vi "Excel Get Last Row (dynamic wrapper).vi"(0 "report in":refnum<class "NI_report.lvclass">, 7 "offset":i32, 11 "error in (no error)":errorcluster, 12 "MS Office parameters":T1) -> (4 "report out":refnum<class "NI_report.lvclass">, 14 "MS Office parameters out":T1, 15 "error out":errorcluster)   [LabVIEW 2020, in "NI_ReportGenerationCore.lvlib"]
uses:
  <vilib>/Utility/NIReport.llb/NI_ReportGenerationCore.lvlib
  <vilib>/Utility/NIReport.llb/NI_report.lvclass
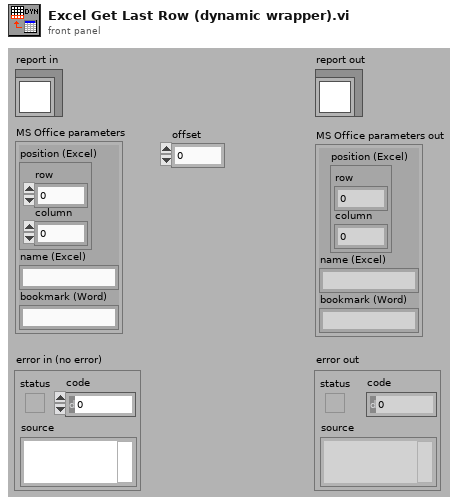
[diagram p1: front panel]
types:
  T1 = cluster{"position (Excel)":cluster{"row":i32, "column":i32}, "name (Excel)":string, "bookmark (Word)":string}
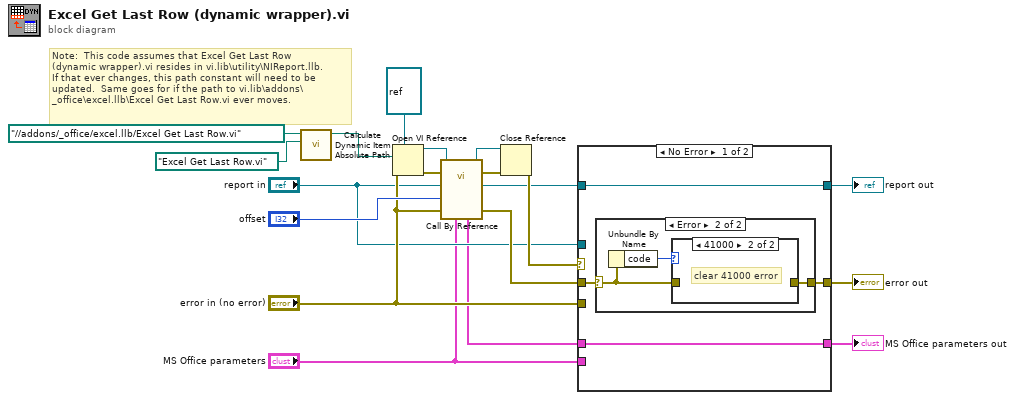
[diagram p0: block diagram]
diagram:
  # "Note:  This code assumes that Excel Get Last Row\n(dynamic wrapper).vi resides in vi.lib\\utility\\NIReport.llb.\nIf that ever changes, this path constant will need to be \nupdated.  Same goes for if the path to vi.lib\\addons\\\n_office\\excel.llb\\Excel Get Last Row.vi ever moves."
  n1 = call <vilib>:"Calculate Dynamic Item Absolute Path.vi"("Compat Built App Relative Path"=path "Excel Get Last Row.vi", "Core Relative Path"=path "../../addons/_office/excel.llb/Excel Get Last Row.vi") -> ("Resulting Absolute Path"=w2:path)  [unwired: 9 out]
  n2 = Open VI Reference(type specifier VI Refnum (for type only)=refnum<vi> refnum ("VI Refnum"), vi path=w2, error in (no error)="error in (no error)") -> (vi reference=w17:refnum<vi>, error out=w19:errorcluster)  [unwired: 3 out]
  n3 = call-by-ref "?"(reference=w17, error in=w19, "report in"="report in", "offset"="offset", 11:"error in (no error)"="error in (no error)", "MS Office parameters"="MS Office parameters") -> (reference out=w16:refnum<vi>, error out=w18:errorcluster, "report out"=w7:refnum<class "NI_report.lvclass">, "MS Office parameters out"=w4:T1, 15:"error out"=w13:errorcluster)  [unwired: 9 in]
  n4 = Close Reference(reference=w16, error in (no error)=w18) -> (error out=w11:errorcluster)
  n5 = case shown="No Error" w11 {
    tunnel: w13 -> [w23 _]
    tunnel: [w22 w31] -> w12
    tunnel: "error in (no error)" -> [_ w31]
    tunnel: "report in" -> [_ w30]
    tunnel: [w21 w30] -> w8
    tunnel: w7 -> [w21 _]
    tunnel: w4 -> [w20 _]
    tunnel: "MS Office parameters" -> [_ w29]
    tunnel: [w20 w29] -> w5
    frame No Error {
      n6 = case shown="Error" w23 {
        selector: w23 -> [w24 w26]
        tunnel: [w24 w25] -> w22
        frame No Error {
        }
        frame Error {
          n7 = Unbundle By Name(w26) -> ("code"=w27:i32)
          n8 = case shown="41000" w27 {
            tunnel: w26 -> [w28 _]
            tunnel: [w28 _] -> w25
            frame Default {
            }
            frame 41000 {
              # "clear 41000 error"
            }
          }
        }
      }
    }
    frame Error {
      # "on error, pass existing inputs"
    }
  }
  "error out" <- w12
  "report out" <- w8
  "MS Office parameters out" <- w5
